vi "WPI_AnalogChannelSetSampleRate.vi"(8 "error in (no error)":errorcluster, 9 "Scan List":T1[](array[typedef]), 10 "Samples Per Second (per channel)":dbl) -> (0 "error out":errorcluster)   [LabVIEW 2017]
doc: "Sets the sample rate for a channel on the controller you specify. The sample rate is the same for each channel on the controller. Use the GetSampleRate VI to return the sample rate of a channel.\n\nThis software is licensed. Open the labview\\readme\\WPI Robotics Library Open Source License.txt file for more information."
uses:
  <vilib>/Rock Robotics/SystemInterfaces/AI/FPGA_AIChannel.ctl
  <vilib>/Rock Robotics/SystemInterfaces/System/FPGA_SystemGet.vi
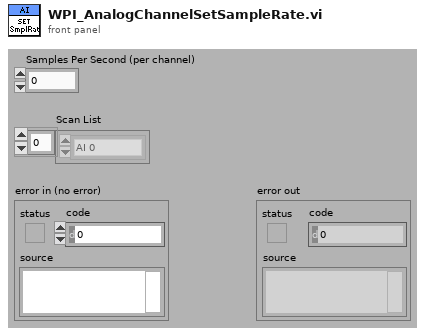
[diagram p1: front panel]
types:
  T1 = typedef "FPGA_AIChannel.ctl" = enum8{"AI 0", "AI 1", "AI 2", "AI 3", "AI MXP 0", "AI MXP 1", "AI MXP 2", "AI MXP 3", "Invalid"}
  T2 = typedef "FPGA_AIDevRef.ctl" = cluster{"DevStatus":errorcluster}
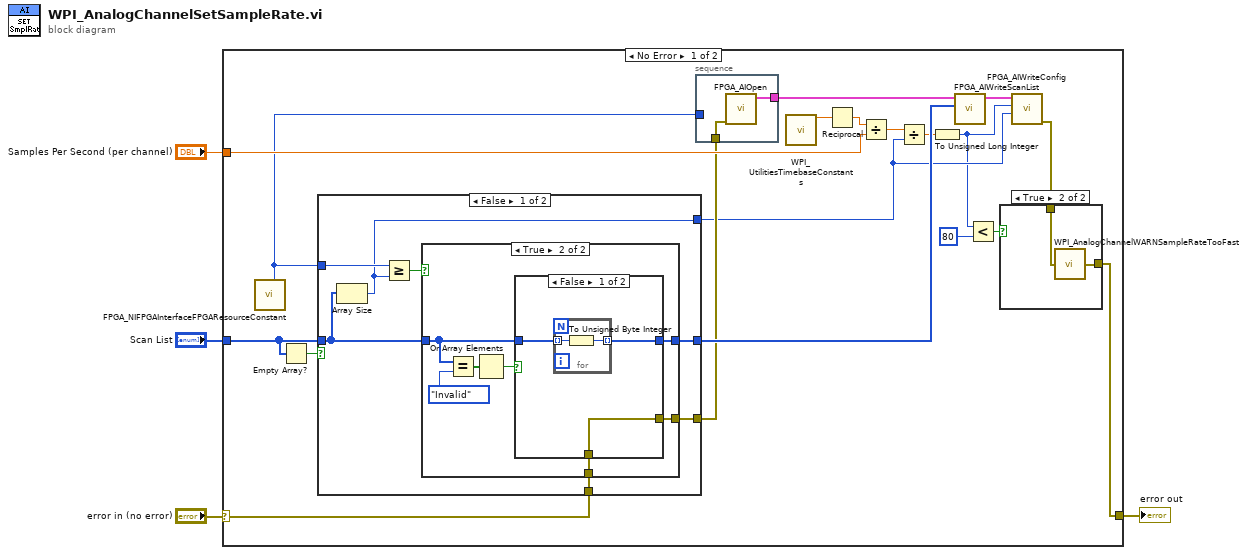
[diagram p0: block diagram]
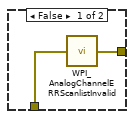
[diagram p3: hidden frame]
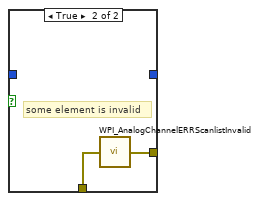
[diagram p4: hidden frame]
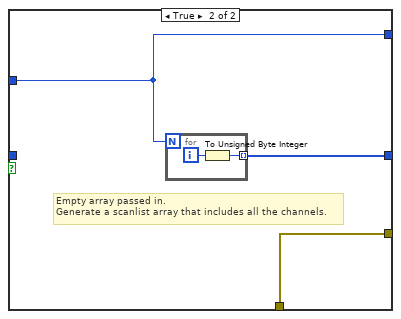
[diagram p5: hidden frame]
diagram:
  n1 = case shown="No Error" "error in (no error)" {
    selector: "error in (no error)" -> [w8 w57]
    tunnel: "Samples Per Second (per channel)" -> [w23 _]
    tunnel: [w9 w57] -> w2
    tunnel: "Scan List" -> [w18 _]
    frame No Error {
      n2 = call <vilib>:"FPGA_NIFPGAInterfaceFPGAResourceConstant.vi"() -> ("NumberOfAIChannels"=w7:u8)  [unwired: 11 out]
      n3 = Empty Array?(array=w18) -> (empty?=w19:bool)
      n4 = case shown="False" w19 {
        tunnel: w7 -> [w33 w53]
        tunnel: [w32 w54] -> w20
        tunnel: w18 -> [w34 _]
        tunnel: [w31 w53] -> w15
        tunnel: [w30 w52] -> w17
        tunnel: w8 -> [w29 w52]
        frame False {
          n5 = Array Size(array=w34) -> (size(s)=w31:i32)
          n6 = Greater Or Equal?(x=w33, y=w31) -> (x >= y?=w35:bool)
          n7 = case shown="True" w35 {
            tunnel: w34 -> [_ w44]
            tunnel: [_ w40] -> w32
            tunnel: [w37 w39] -> w30
            tunnel: w29 -> [w36 w38]
            frame False {
              n8 = call <vilib>:"WPI_AnalogChannelERRScanlistInvalid.vi"("error in (no error)"=w36) -> ("error out"=w37:errorcluster)
            }
            frame True {
              n9 = Equal?(x=w44, y=FPGA_AIChannel."Invalid" ("Channel")) -> (x = y?=w42:bool[])
              n10 = Or Array Elements(Boolean array=w42) -> (logical OR=w41:bool)
              n11 = case shown="False" w41 {
                tunnel: w44 -> [w47 _]
                tunnel: [w46 _] -> w40
                tunnel: [w45 w51] -> w39
                tunnel: w38 -> [w45 w50]
                frame False {
                  n12 = for {
                    tunnel: w47 -> [w49] mode=indexing
                    tunnel: [w48] -> w46 mode=indexing
                    n13 = To Unsigned Byte Integer(number=w49) -> (unsigned 8bit integer=w48:u8)
                  }
                }
                frame True {
                  # "some element is invalid"
                  n14 = call <vilib>:"WPI_AnalogChannelERRScanlistInvalid.vi"("error in (no error)"=w50) -> ("error out"=w51:errorcluster)
                }
              }
            }
          }
        }
        frame True {
          # "Empty array passed in.\nGenerate a scanlist array that includes all the channels."
          n15 = for {
            N: w53 -> [_]
            tunnel: [w55] -> w54 mode=indexing
            i -> [w56]
            n16 = To Unsigned Byte Integer(number=w56) -> (unsigned 8bit integer=w55:u8)
          }
        }
      }
      n17 = stacked-sequence {
        tunnel: w17 -> [w25]
        tunnel: [w24] -> w16
        tunnel: w7 -> [_]
        frame #0 {
          n18 = call <vilib>:"FPGA_AIOpen.vi"("error in (no error)"=w25) -> ("AI Reference out"=w24:T2)  [unwired: 2 in, 8 out]
        }
      }
      n19 = call <vilib>:"WPI_UtilitiesTimebaseConstants.vi"() -> ("40 MHz FPGA clock"=w6:dbl)  [unwired: 13 in, 2 out]
      n20 = Reciprocal(x=w6) -> (1/x=w5:dbl)
      n21 = Divide(x=w5, y=w23) -> (x/y=w22:dbl)
      n22 = Divide(x=w22, y=w15) -> (x/y=w13:dbl)
      n23 = To Unsigned Long Integer(number=w13) -> (unsigned 32bit integer=w11:u32)
      n24 = call <vilib>:"FPGA_AIWriteScanList.vi"("Scan List"=w20, "AI Reference"=w16) -> ("AI Reference"=w21:T2)  [unwired: 1 in, 8 out]
      n25 = Less?(x=w11, y=u32 80) -> (x < y?=w14:bool)
      n26 = call <vilib>:"FPGA_AIWriteConfig.vi"("Scan Size"=w15, "Convert Rate"=w11, "AI Reference"=w21) -> ("error out"=w10:errorcluster)  [unwired: 1 in, 7 out]
      n27 = case shown="True" w14 {
        tunnel: [w26 w28] -> w9
        tunnel: w10 -> [w26 w27]
        frame False {
        }
        frame True {
          n28 = call <vilib>:"WPI_AnalogChannelWARNSampleRateTooFast.vi"("error in (no error)"=w27) -> ("error out"=w28:errorcluster)
        }
      }
    }
    frame Error {
    }
  }
  "error out" <- w2
